vi "test Error on Last Ack.vi"(8 "error in (no error)":errorcluster, 11 "TestCase in":refnum<class "Test Nested Endpoint Transmit Failure.lvclass">) -> (0 "error out":errorcluster, 3 "TestCase out":refnum<class "Test Nested Endpoint Transmit Failure.lvclass">)   [LabVIEW 2020, in "Test Nested Endpoint Transmit Failure.lvclass"]
uses:
  Test Nested Endpoint Transmit Failure.lvclass
  <vilib>/addons/_JKI Toolkits/VI Tester/TestCase.llb/TestCase.lvclass
  <vilib>/ActorFramework/Message Queue/Message Queue.lvclass
  <vilib>/ActorFramework/Message Dequeuer/Message Dequeuer.lvclass
  <vilib>/ActorFramework/LastAck/Last Ack.lvclass
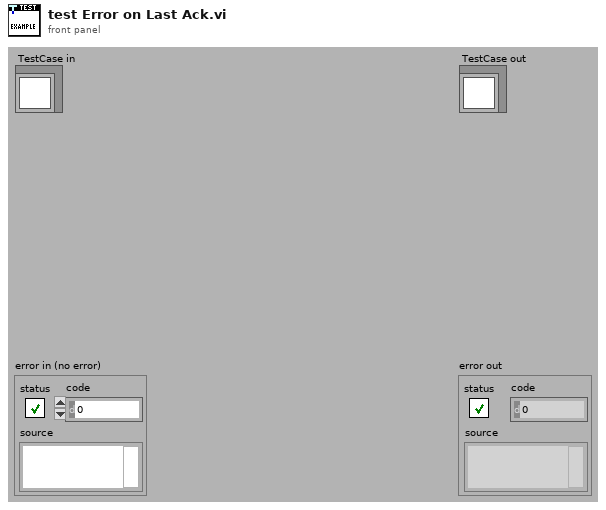
[diagram p1: front panel]
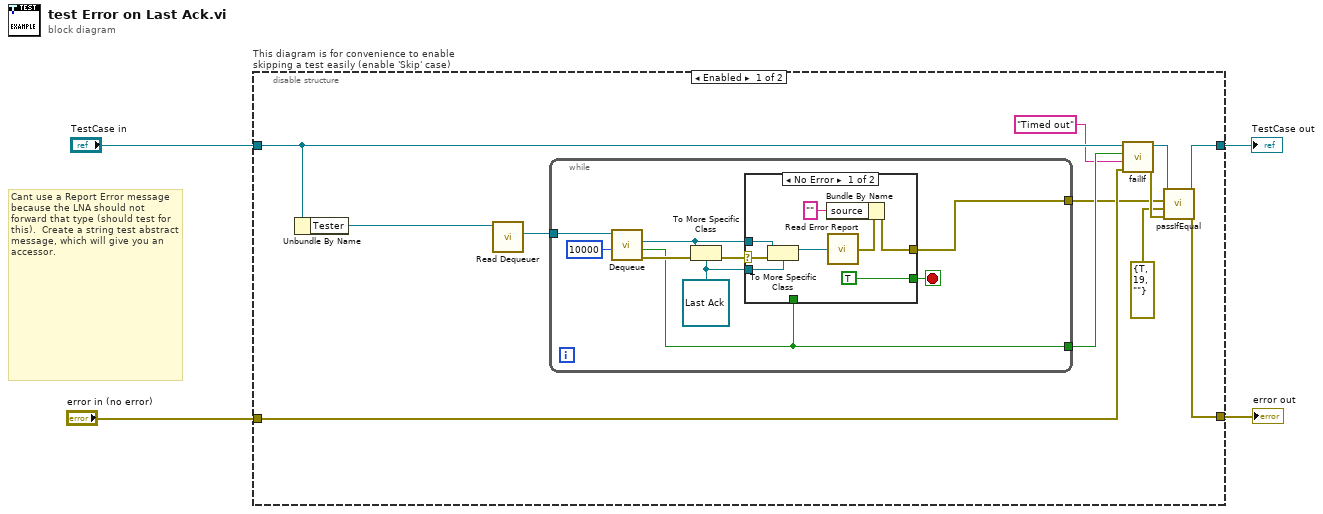
[diagram p0: block diagram]
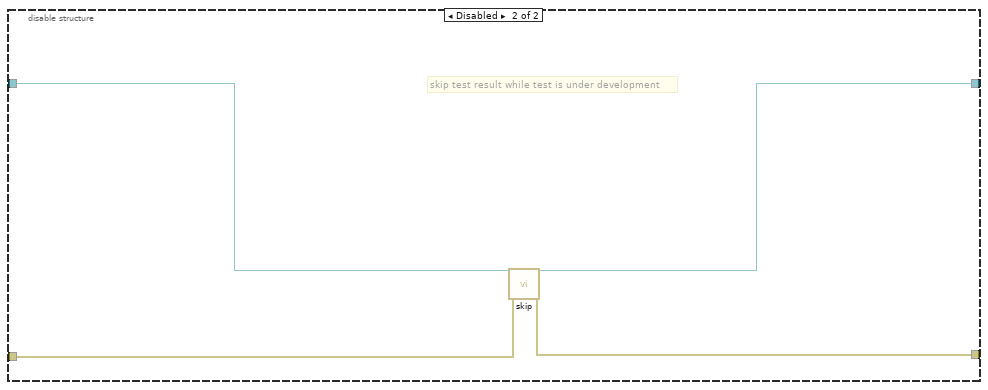
[diagram p3: hidden frame]
diagram:
  # "Cant use a Report Error message because the LNA should not forward that type (should test for this).  Create a string test abstract message, which will give you an accessor."
  n1 = disable-structure "This diagram is for convenience to enable skipping a test easily (enable 'Skip' case)" shown="Enabled" {
    disable-tunnel: "TestCase in" -> [w12 w38]
    disable-tunnel: [w16 w36] -> w1
    disable-tunnel: [w15 w37] -> w3
    disable-tunnel: "error in (no error)" -> [w7 w35]
    frame Enabled {
      n2 = Unbundle By Name(w12) -> ("Tester"=w13:refnum<class "Message Queue.lvclass">)
      n3 = call <vilib>:"Read Dequeuer.vi"("Message Queue"=w13) -> ("Message Dequeuer"=w14:refnum<class "Message Dequeuer.lvclass">)  [unwired: 10 in]
      n4 = while {
        tunnel: w14 -> [w25]
        tunnel: [w17] -> w10
        tunnel: [w18] -> w6
        stop <- w19 stop-if-true
        w20 = refnum<class "Last Ack.lvclass"> refnum ("Last Ack")
        n5 = call <vilib>:"Dequeue.vi"("timeout in ms (-1)"=10000, "Message Dequeuer in"=w25) -> ("error out"=w23:errorcluster, "timed out?"=w17:bool, "Message"=w21:refnum<class "Message.lvclass">)  [unwired: 5 in, 2 out]
        n6 = To More Specific Class(target class=w20, reference=w21, error in=w23) -> (error out=w22:errorcluster)  [unwired: 1 out]
        n7 = case shown="No Error" w22 {
          selector: w22 -> [w33 _]
          tunnel: w21 -> [w32 _]
          tunnel: w20 -> [w31 _]
          tunnel: [w27 _] -> w18
          tunnel: [TRUE w34] -> w19
          tunnel: w17 -> [_ w34]
          frame No Error {
            n8 = To More Specific Class(target class=w31, reference=w32, error in=w33) -> (specific class reference=w30:refnum<class "Last Ack.lvclass">)  [unwired: 1 out]
            n9 = call <vilib>:"Read Error Report.vi"("Last Ack"=w30) -> ("error report"=w29:errorcluster)
            n10 = Bundle By Name(cluster=w29, "source"="") -> (w27:errorcluster)
          }
          frame Error {
          }
        }
      }
      n11 = call-dynamic "failIf.vi"("error in (no error)"=w7, "message (\"\")"="Timed out" ("message (\"\")"), "fail"=w10, "TestCase in"=w12) -> ("error out"=w9:errorcluster, "TestCase out"=w11:refnum<class "Test Nested Endpoint Transmit Failure.lvclass">)  [unwired: 6 in]
      n12 = call-dynamic "passIfEqual.vi"("error in (no error)"=w9, "y"=errorcluster {"status"=TRUE, "code"=19, "source"=""} ("error report"), "x"=w6, "TestCase in"=w11) -> ("error out"=w15:errorcluster, "TestCase out"=w16:refnum<class "Test Nested Endpoint Transmit Failure.lvclass">)  [unwired: 6 in]
    }
    frame Disabled {
      # "skip test result while test is under development"
      n13 = call <vilib>:"skip.vi"("error in (no error)"=w35, "TestCase in"=w38) -> ("error out"=w37:errorcluster, "TestCase out"=w36:refnum<class "Test Nested Endpoint Transmit Failure.lvclass">)  [unwired: 8 in]
    }
  }
  "error out" <- w3
  "TestCase out" <- w1
